vi "Defer Panel Updates.vi"(6 "Set Defer Panel Updates? [T]":bool=TRUE, 7 "VI Refnum":refnum<vi>, 8 "error in (no error)":errorcluster, 10 "Defer Panel Updates? [T]":bool=TRUE) -> (0 "error out":errorcluster)   [LabVIEW 2021, in "IObject.lvclass"]
uses:
  IObject.lvclass
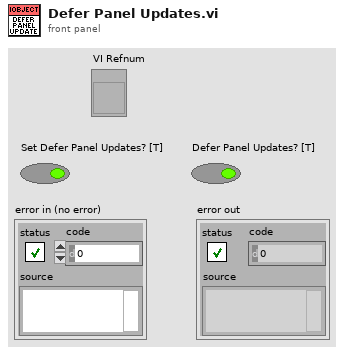
[diagram p1: front panel]
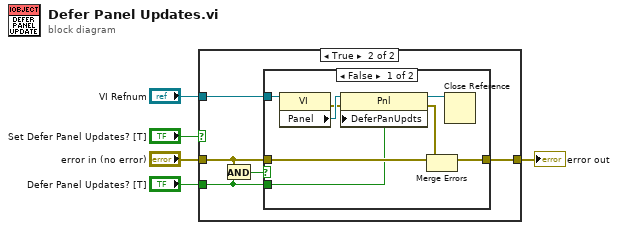
[diagram p0: block diagram]
diagram:
  n1 = case shown="True" "Set Defer Panel Updates? [T]" {
    tunnel: "error in (no error)" -> [w6 w9]
    tunnel: "VI Refnum" -> [_ w11]
    tunnel: [w6 w10] -> w2
    tunnel: "Defer Panel Updates? [T]" -> [_ w7]
    frame False {
    }
    frame True {
      n2 = And(x=w9, y=w7) -> (x .and. y?=w8:bool)
      n3 = case shown="False" w8 {
        tunnel: w11 -> [w19 _]
        tunnel: w7 -> [w12 _]
        tunnel: w9 -> [w17 w20]
        tunnel: [w16 w20] -> w10
        frame False {
          n4 = property class="VI"(reference=w19) -> (error out=w14:errorcluster, "Panel"=w18:refnum<vi>)  [unwired: 1 in, 1 out]
          n5 = property class="Pnl"(reference=w18, error in=w14, "DeferPanUpdts"=w12) -> (reference out=w13:refnum<vi>, error out=w15:errorcluster)
          n6 = Merge Errors(w17, w15) -> (w16:errorcluster)
          n7 = Close Reference(reference=w13) -> ()  [unwired: 1 in, 1 out]
        }
        frame True {
        }
      }
    }
  }
  "error out" <- w2
